vi "Write_MaxTimeout(s).vi"(8 "error in (no error)":errorcluster, 10 "Max Timeout(s)":dbl, 11 "Subsystem in":refnum<class "Subsystem.lvclass">) -> (0 "error out":errorcluster, 3 "Subsystem out":refnum<class "Subsystem.lvclass">)   [LabVIEW 2017, in "Subsystem.lvclass"]
uses:
  Subsystem.lvclass
  Subsystem.lvclass/Subsystem.ctl
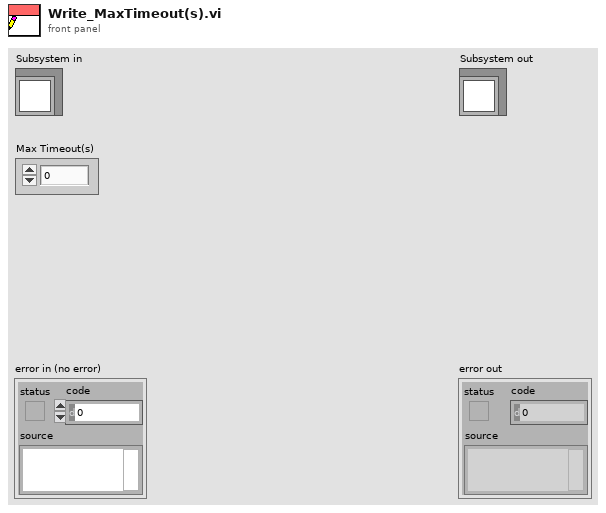
[diagram p1: front panel]
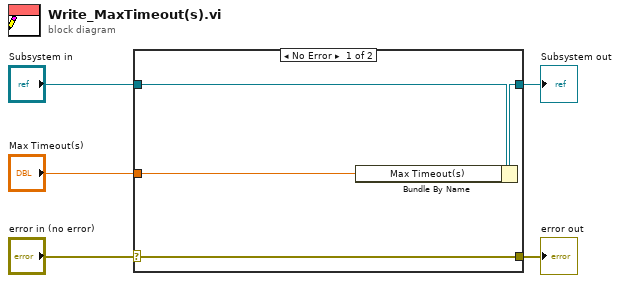
[diagram p0: block diagram]
diagram:
  n1 = case shown="No Error" "error in (no error)" {
    selector: "error in (no error)" -> [w9 w10]
    tunnel: [w9 w10] -> w4
    tunnel: [w7 w11] -> w2
    tunnel: "Subsystem in" -> [w8 w11]
    tunnel: "Max Timeout(s)" -> [w6 _]
    frame No Error {
      n2 = Bundle By Name(cluster=w8, "Max Timeout(s)"=w6) -> (w7:refnum<class "Subsystem.lvclass">)
    }
    frame Error {
    }
  }
  "error out" <- w4
  "Subsystem out" <- w2
